vi "tictoc.vi"(0 "Value":dbl format="%.2f", 1 "Value 2":dbl format="%.2f") -> (2 "sec":dbl format="%.2f", 3 "min":dbl format="%.2f", 4 "hour":dbl format="%.2f")   [LabVIEW 2010]
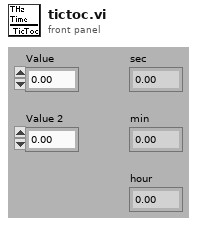
[diagram p1: front panel]
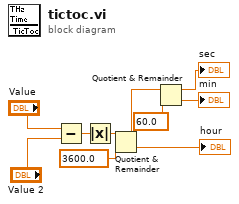
[diagram p0: block diagram]
diagram:
  n1 = Subtract(x="Value", y="Value 2") -> (x-y=w2:dbl)
  n2 = Absolute Value(x=w2) -> (abs(x)=w1:dbl)
  n3 = Quotient & Remainder(x=w1, y=3600.0) -> (x-y*floor(x/y)=w6:dbl, floor(x/y)=→"hour":dbl)
  n4 = Quotient & Remainder(x=w6, y=60.0) -> (x-y*floor(x/y)=→"sec":dbl, floor(x/y)=→"min":dbl)
